vi "wd_length_create.vi"(8 "error in (no error)":errorcluster, 9 "data type":T7, 10 "size":u64, 11 "meta in":T1={"TargetFile"=path "", "StreamMode"=enum."File", "Append?"=FALSE, "ChunkSize"=0, "TimeColumnMode"=enum."Empty", "TimestampFormat"="", "AbsoluteTime?"=FALSE, "FileAttribute "={"Creator"="", "Title"="", "SheetName"=""}, "Column"=[], "FileRef"=refnum, "MemoryRef"=[], "RecordInfo"=[], " ChannelPreviousInfo"=[], "ChannelFirstRecord"=[], "PredefinedFormattedValueLength"=20, "DiskTemplate"={"XMLRef"=[refnum, refnum, refnum, refnum, refnum, refnum], "ZipPath"=path "", "MetaFile"={"Ref"=refnum, "NextRow"=0, "NextPosition"=0, "Block"=[]}, "TempFolder"=path ""}}) -> (0 "error out":errorcluster, 3 "meta out":T1={"TargetFile"=path "", "StreamMode"=enum."File", "Append?"=FALSE, "ChunkSize"=0, "TimeColumnMode"=enum."Empty", "TimestampFormat"="", "AbsoluteTime?"=FALSE, "FileAttribute "={"Creator"="", "Title"="", "SheetName"=""}, "Column"=[], "FileRef"=refnum, "MemoryRef"=[], "RecordInfo"=[], " ChannelPreviousInfo"=[], "ChannelFirstRecord"=[], "PredefinedFormattedValueLength"=20, "DiskTemplate"={"XMLRef"=[refnum, refnum, refnum, refnum, refnum, refnum], "ZipPath"=path "", "MetaFile"={"Ref"=refnum, "NextRow"=0, "NextPosition"=0, "Block"=[]}, "TempFolder"=path ""}})   [LabVIEW 2017, in "NI_ExcelFile.lvlib"]
uses:
  <vilib>/express/express shared/NI_ExcelFile/NI_ExcelFile.lvlib
  <vilib>/express/express shared/NI_ExcelFile/Ctrls/DataType.ctl
  <vilib>/express/express shared/NI_ExcelFile/Ctrls/MainData.ctl
  <vilib>/express/express shared/NI_ExcelFile/Ctrls/StreamMode.ctl
  <vilib>/express/express shared/NI_ExcelFile/Ctrls/TimeColumnMode.ctl
  <vilib>/express/express shared/NI_ExcelFile/Ctrls/FileAttribute.ctl
  <vilib>/express/express shared/NI_ExcelFile/Ctrls/Columns.ctl
  <vilib>/express/express shared/NI_ExcelFile/Ctrls/ColumnInfo.ctl
  <vilib>/express/express shared/NI_ExcelFile/Ctrls/wd_recordInfo.ctl
  <vilib>/express/express shared/NI_ExcelFile/Ctrls/disk_TemplateFile.ctl
  <vilib>/express/express shared/NI_ExcelFile/Ctrls/meta_file.ctl
  <vilib>/express/express shared/NI_ExcelFile/Ctrls/meta_Block.ctl
  <vilib>/express/express shared/NI_ExcelFile/Ctrls/meta_BlockType.ctl
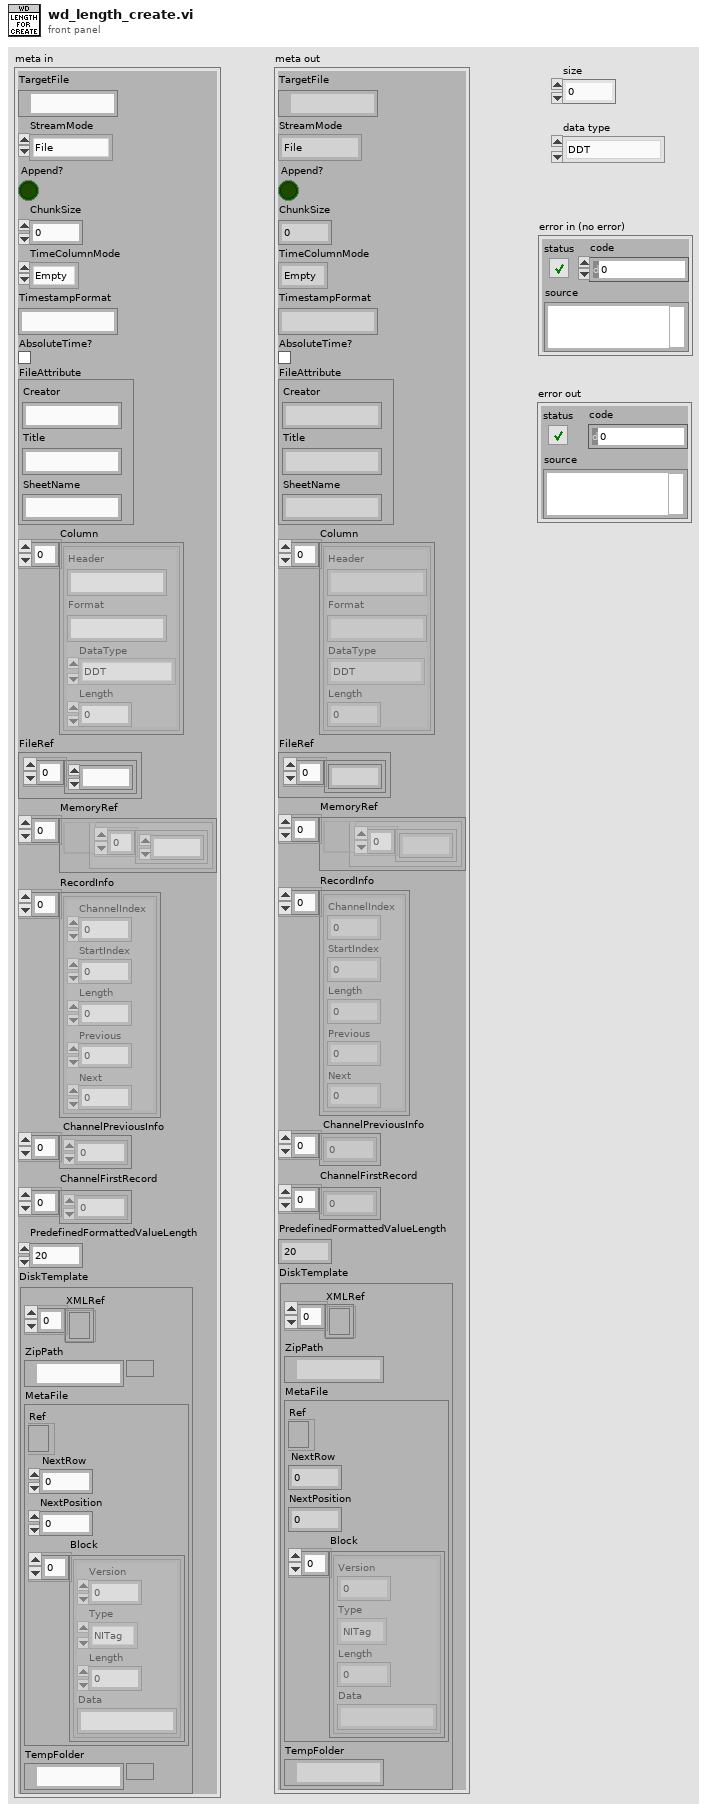
[diagram p1: front panel]
types:
  T1 = typedef "NI_ExcelFile.lvlib/MainData.ctl" = cluster{"TargetFile":path, "StreamMode":T2, "Append?":bool, "ChunkSize":u64, "TimeColumnMode":T3, "TimestampFormat":string, "AbsoluteTime?":bool, "FileAttribute ":T4, "Column":T5, "FileRef":refnum<k1>, "MemoryRef":refnum<data-value>[], "RecordInfo":T8[], " ChannelPreviousInfo":u32[], "ChannelFirstRecord":u32[], "PredefinedFormattedValueLength":i64, "DiskTemplate":T9}
  T2 = typedef "NI_ExcelFile.lvlib/StreamMode.ctl" = enum16{"File", "Memory"}
  T3 = typedef "NI_ExcelFile.lvlib/TimeColumnMode.ctl" = enum16{"Empty", "OnePerCh", "One"}
  T4 = typedef "NI_ExcelFile.lvlib/FileAttribute.ctl" = cluster{"Creator":string, "Title":string, "SheetName":string}
  T5 = typedef "NI_ExcelFile.lvlib/Columns.ctl" = T6[]
  T6 = typedef "NI_ExcelFile.lvlib/ColumnInfo.ctl" = cluster{"Header":string, "Format":string, "DataType":T7, "Length":u64}
  T7 = typedef "NI_ExcelFile.lvlib/DataType.ctl" = enum16{"DDT", "WFM", "Array of STR", "Array of DBL", "Array of I8", "Array of I16", "Array of I32", "Array of I64", "Array of SGL", "Array of U8", "Array of U16", "Array of U32", "Array of U64", "Array of Time"}
  T8 = typedef "NI_ExcelFile.lvlib/wd_recordInfo.ctl" = cluster{"ChannelIndex":u32, "StartIndex":u64, "Length":u64, "Previous":i32, "Next":i32}
  T9 = typedef "NI_ExcelFile.lvlib/disk_TemplateFile.ctl" = cluster{"XMLRef":refnum<file>[], "ZipPath":path, "MetaFile":T10, "TempFolder":path}
  T10 = typedef "NI_ExcelFile.lvlib/meta_file.ctl" = cluster{"Ref":refnum<file>, "NextRow":i32, "NextPosition":i64, "Block":T11[]}
  T11 = typedef "NI_ExcelFile.lvlib/meta_Block.ctl" = cluster{"Version":u16, "Type":T12, "Length":i32, "Data":string}
  T12 = typedef "NI_ExcelFile.lvlib/meta_BlockType.ctl" = enum16{"NITag", "File", "Column"}
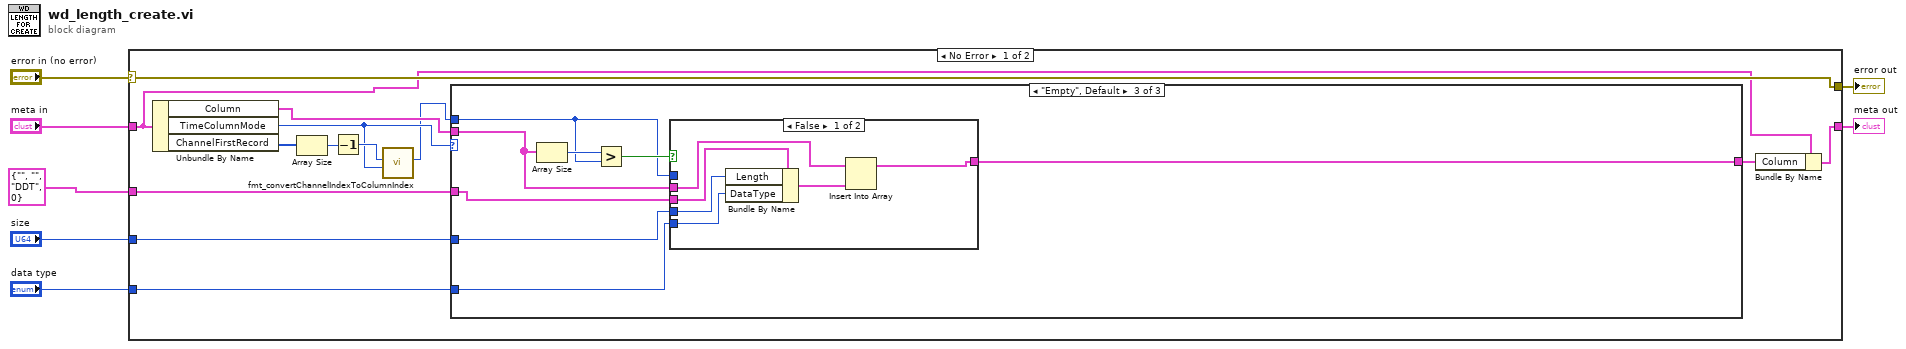
[diagram p0: block diagram]
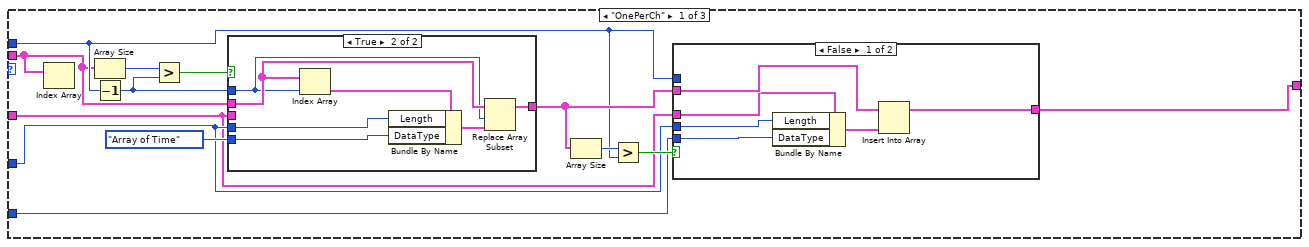
[diagram p2: hidden frame]
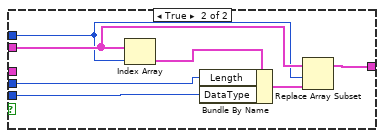
[diagram p3: hidden frame]
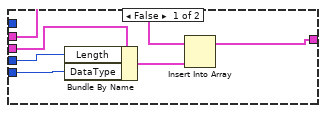
[diagram p4: hidden frame]
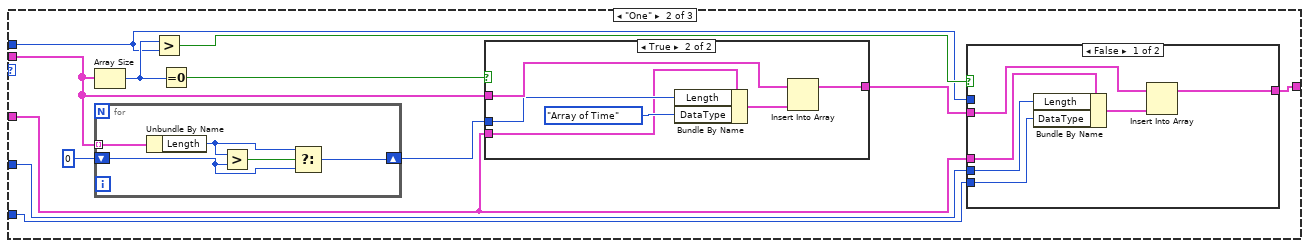
[diagram p5: hidden frame]
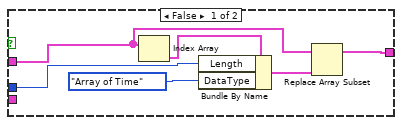
[diagram p6: hidden frame]
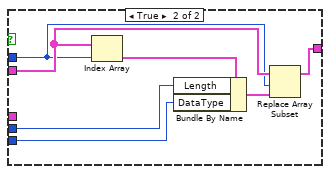
[diagram p7: hidden frame]
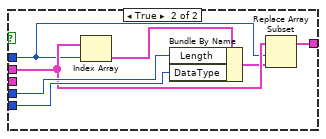
[diagram p8: hidden frame]
diagram:
  n1 = case shown="No Error" "error in (no error)" {
    selector: "error in (no error)" -> [w12 w123]
    tunnel: "size" -> [w20 _]
    tunnel: [w18 w124] -> w6
    tunnel: "data type" -> [w16 _]
    tunnel: "meta in" -> [w8 w124]
    tunnel: [w12 w123] -> w2
    tunnel: T6 {"Header"="", "Format"="", "DataType"=enum."DDT", "Length"=0} ("element") -> [w13 _]
    frame No Error {
      n2 = Unbundle By Name(w8) -> ("Column"=w19:T5, "TimeColumnMode"=w10:T3, "ChannelFirstRecord"=w15:u32[])
      n3 = Array Size(array=w15) -> (size(s)=w14:i32)
      n4 = Decrement(x=w14) -> (x-1=w11:i32)
      n5 = call <vilib>:"fmt_convertChannelIndexToColumnIndex.vi"("TimeColumnMode"=w10, "channel index"=w11) -> ("data column index"=w9:i32)  [unwired: 8 in, 1 out]
      n6 = case shown="\"Empty\", Default" w10 {
        tunnel: [w27 w67 w107] -> w17
        tunnel: w19 -> [w22 w62 w104]
        tunnel: w20 -> [w25 w66 w106]
        tunnel: w16 -> [w24 w65 w105]
        tunnel: w9 -> [w23 w61 w103]
        tunnel: w13 -> [w21 w60 w102]
        frame "OnePerCh" {
          n7 = Index Array(array=w22) -> ()  [unwired: 1 in, 1 out]
          n8 = Array Size(array=w22) -> (size(s)=w33:i32)
          n9 = Decrement(x=w23) -> (x-1=w31:i32)
          n10 = Greater?(x=w33, y=w31) -> (0:w32:bool)
          n11 = case shown="True" w32 {
            tunnel: w22 -> [w52 w56]
            tunnel: w31 -> [_ w55]
            tunnel: [w51 w59] -> w28
            tunnel: DataType."Array of Time" ("Column DataType") -> [w50 w58]
            tunnel: w25 -> [w49 w57]
            tunnel: w21 -> [w47 _]
            frame False {
              n12 = Bundle By Name(cluster=w47, "Length"=w49, "DataType"=w50) -> (w48:T6)
              n13 = Insert Into Array(array=w52, new element=w48) -> (w51:T5)  [unwired: 1 in]
            }
            frame True {
              n14 = Index Array(array=w56, index=w55) -> (element=w54:T6)
              n15 = Bundle By Name(cluster=w54, "Length"=w57, "DataType"=w58) -> (w53:T6)
              n16 = Replace Array Subset(array=w56, new element=w53, index=w55) -> (w59:T5)
            }
          }
          n17 = Array Size(array=w28) -> (size(s)=w30:i32)
          n18 = Greater?(x=w30, y=w23) -> (0:w29:bool)
          n19 = case shown="False" w29 {
            tunnel: w28 -> [w39 w45]
            tunnel: [w38 w46] -> w27
            tunnel: w23 -> [_ w44]
            tunnel: w25 -> [w37 w42]
            tunnel: w24 -> [w36 w41]
            tunnel: w21 -> [w34 _]
            frame False {
              n20 = Bundle By Name(cluster=w34, "Length"=w37, "DataType"=w36) -> (w35:T6)
              n21 = Insert Into Array(array=w39, new element=w35) -> (w38:T5)  [unwired: 1 in]
            }
            frame True {
              n22 = Index Array(array=w45, index=w44) -> (element=w43:T6)
              n23 = Bundle By Name(cluster=w43, "Length"=w42, "DataType"=w41) -> (w40:T6)
              n24 = Replace Array Subset(array=w45, new element=w40, index=w44) -> (w46:T5)
            }
          }
        }
        frame "One" {
          n25 = Array Size(array=w62) -> (size(s)=w63:i32)
          n26 = for {
            shift-right: [w99] -> w70
            shift-left: u64 0 -> [w100]
            tunnel: w62 -> [w98] mode=indexing
            n27 = Unbundle By Name(w98) -> ("Length"=w97:u64)
            n28 = Greater?(x=w97, y=w100) -> (0:w101:bool)
            n29 = Select(t=w97, s=w101, f=w100) -> (s? t:f=w99:u64)
          }
          n30 = Greater?(x=w63, y=w61) -> (0:w69:bool)
          n31 = Equal To 0?(x=w63) -> (x = 0?=w64:bool)
          n32 = case shown="True" w64 {
            tunnel: w70 -> [w77 w82]
            tunnel: [w74 w79] -> w68
            tunnel: w62 -> [w73 w83]
            tunnel: w60 -> [_ w78]
            frame False {
              n33 = Index Array(array=w73) -> (element=w72:T6)  [unwired: 1 in]
              n34 = Bundle By Name(cluster=w72, "Length"=w77, "DataType"=DataType."Array of Time" ("Column DataType")) -> (w75:T6)
              n35 = Replace Array Subset(array=w73, new element=w75) -> (w74:T5)  [unwired: 1 in]
            }
            frame True {
              n36 = Bundle By Name(cluster=w78, "Length"=w82, "DataType"=DataType."Array of Time" ("Column DataType")) -> (w80:T6)
              n37 = Insert Into Array(array=w83, new element=w80) -> (w79:T5)  [unwired: 1 in]
            }
          }
          n38 = case shown="False" w69 {
            tunnel: w68 -> [w88 w93]
            tunnel: w61 -> [_ w90]
            tunnel: [w89 w96] -> w67
            tunnel: w66 -> [w87 w95]
            tunnel: w65 -> [w86 w94]
            tunnel: w60 -> [w84 _]
            frame False {
              n39 = Bundle By Name(cluster=w84, "Length"=w87, "DataType"=w86) -> (w85:T6)
              n40 = Insert Into Array(array=w88, new element=w85) -> (w89:T5)  [unwired: 1 in]
            }
            frame True {
              n41 = Index Array(array=w93, index=w90) -> (element=w92:T6)
              n42 = Bundle By Name(cluster=w92, "Length"=w95, "DataType"=w94) -> (w91:T6)
              n43 = Replace Array Subset(array=w93, new element=w91, index=w90) -> (w96:T5)
            }
          }
        }
        frame "Empty", Default {
          n44 = Array Size(array=w104) -> (size(s)=w109:i32)
          n45 = Greater?(x=w109, y=w103) -> (0:w108:bool)
          n46 = case shown="False" w108 {
            tunnel: w104 -> [w114 w119]
            tunnel: w103 -> [_ w116]
            tunnel: [w115 w122] -> w107
            tunnel: w106 -> [w113 w121]
            tunnel: w105 -> [w112 w120]
            tunnel: w102 -> [w110 _]
            frame False {
              n47 = Bundle By Name(cluster=w110, "Length"=w113, "DataType"=w112) -> (w111:T6)
              n48 = Insert Into Array(array=w114, new element=w111) -> (w115:T5)  [unwired: 1 in]
            }
            frame True {
              n49 = Index Array(array=w119, index=w116) -> (element=w118:T6)
              n50 = Bundle By Name(cluster=w118, "Length"=w121, "DataType"=w120) -> (w117:T6)
              n51 = Replace Array Subset(array=w119, new element=w117, index=w116) -> (w122:T5)
            }
          }
        }
      }
      n52 = Bundle By Name(cluster=w8, "Column"=w17) -> (w18:T1)
    }
    frame Error {
    }
  }
  "meta out" <- w6
  "error out" <- w2
